vi "Configure Secured TCP Server.vi"(4 "Read Mode (Immediate)":T1(ring)=enum."Immediate", 5 "password":string, 6 "timeout ms":i32=5000, 7 "Server private key":path, 8 "error in (no error)":errorcluster, 9 "Server X.509 Certificate":path, 10 "remote port (443)":u16=443, 11 "address (localhost)":string="localhost") -> (0 "error out":errorcluster, 2 "Ready for SSL":bool, 3 "Secured TCP Connection":refnum<class "Connection.TCP-TLS.lvclass">)   [LabVIEW 2020, in "Connection.TCP-TLS.lvclass"]
uses:
  Connection.TCP-TLS.lvclass
  Connection.TCP-TLS.lvclass/Connection.TCP-TLS.ctl
  <vilib>/LabVIEW Open Source Project/MQTT TCP Connection/MQTT_TCP/Connection/TCPConnection.lvclass
  <vilib>/LabVIEW Open Source Project/Connection/Connection/Connection.lvclass
  C:/Program Files (x86)/National Instruments/LabVIEW 2020/vi.lib/LabVIEW Open Source Project/MQTT TCP Connection/MQTT_TCP/Connection/TCPConnection.lvclass
  C:/Program Files (x86)/National Instruments/LabVIEW 2020/vi.lib/LabVIEW Open Source Project/MQTT Connection/MQTT_Connection/Connection/Connection.lvclass
  C:/Program Files (x86)/National Instruments/LabVIEW 2020/vi.lib/LabVIEW Open Source Project/Connection/Connection/Connection.lvclass
  C:/Repositories/LVOS/MQTT-Connection-SecuredTCP/source/Connection.SecuredTCP/Connection.TCP-TLS.lvclass
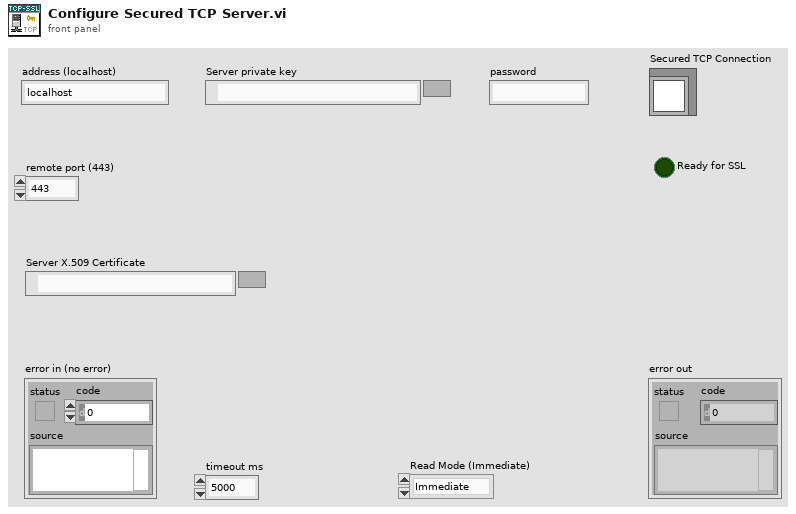
[diagram p1: front panel]
types:
  T1 = enum16{"Standard", "Buffered", "CRLF", "Immediate"}
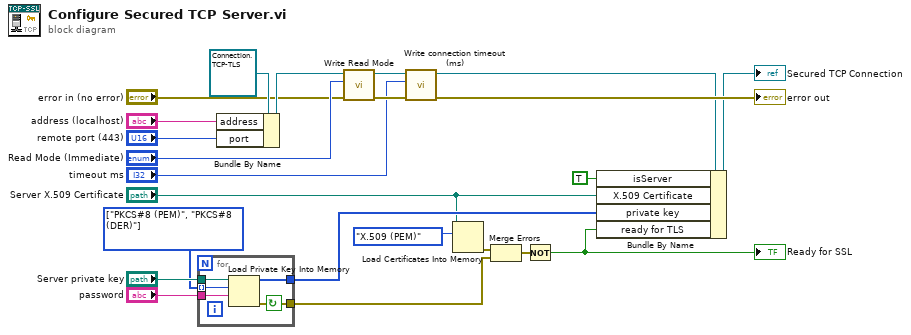
[diagram p0: block diagram]
diagram:
  w10 = enum32{"PKCS#8 (PEM)", "PKCS#8 (DER)"}[] [enum."PKCS#8 (PEM)", enum."PKCS#8 (DER)"] items=["PKCS#8 (PEM)", "PKCS#8 (DER)"]
  n1 = for {
    tunnel: "Server private key" -> [w28]
    tunnel: "password" -> [w27]
    tunnel: w10 -> [w26] mode=indexing
    tunnel: [w25] -> w5
    tunnel: [w24] -> w8
    stop <- w24 continue-if-true
    n2 = Load Private Key Into Memory(9:w27, 10:w26, 11:w28) -> (0:w24:errorcluster, 3:w25:u8[])  [unwired: 1 in]
  }
  n3 = Bundle By Name(cluster=refnum<class "Connection.TCP-TLS.lvclass"> refnum ("Connection.TCP-TLS in"), "address"="address (localhost)", "port"="remote port (443)") -> (w19:refnum<class "Connection.TCP-TLS.lvclass">)
  n4 = call <vilib>:"Write Read Mode.vi"("error in (no error)"="error in (no error)", "Read Mode"="Read Mode (Immediate)", "TCPConnection in"=w19) -> ("error out"=w18:errorcluster, "TCPConnection"=w20:refnum<class "Connection.TCP-TLS.lvclass">)  [unwired: 7 in]
  n5 = call <vilib>:"Write connection timeout (ms).vi"("error in (no error)"=w18, "connection timeout (ms)"="timeout ms", "Connection in"=w20) -> ("error out"=→"error out":errorcluster, "Connection out"=w6:refnum<class "Connection.TCP-TLS.lvclass">)  [unwired: 7 in]
  n6 = Load Certificates Into Memory(10:enum32{"X.509 (PEM)"}."X.509 (PEM)" ("format"), 11:"Server X.509 Certificate") -> (0:w9:errorcluster)  [unwired: 1 in, 1 out]
  n7 = Merge Errors(w9, w8) -> (w7:errorcluster)
  n8 = Not(x=w7) -> (.not. x?=w2:bool)
  "Ready for SSL" <- w2
  n9 = Bundle By Name(cluster=w6, "isServer"=TRUE, "X.509 Certificate"="Server X.509 Certificate", "private key"=w5, "ready for TLS"=w2) -> (→"Secured TCP Connection":refnum<class "Connection.TCP-TLS.lvclass">)
